vi "Initialize Attributes Core.vi"(8 "error in (no error)":errorcluster, 10 "Attribute Data":variant, 11 "BNT_DSCXYGraph in":refnum<class "BNT_DSCXYGraph.lvclass">) -> (0 "error out":errorcluster, 2 "MandatoryParameters":cluster{"Parameter":string, "found?":bool}[](array[cluster]), 3 "BNT_DSCXYGraph out":refnum<class "BNT_DSCXYGraph.lvclass">)   [LabVIEW 2018, in "BNT_DSCXYGraph.lvlib" / "BNT_DSCXYGraph.lvclass"]
doc: "Initialize object attribute.\n\nUnique resources should be allocated elsewhere!"
uses:
  BNT_DSCXYGraph.lvclass
  BNT_DSCXYGraph.lvclass/BNT_DSCXYGraph.ctl
  CSPP_Core/Actors/CSPP_GUIActor/CSPP_GUIActor.lvclass
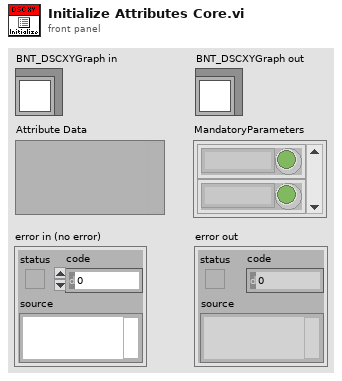
[diagram p1: front panel]
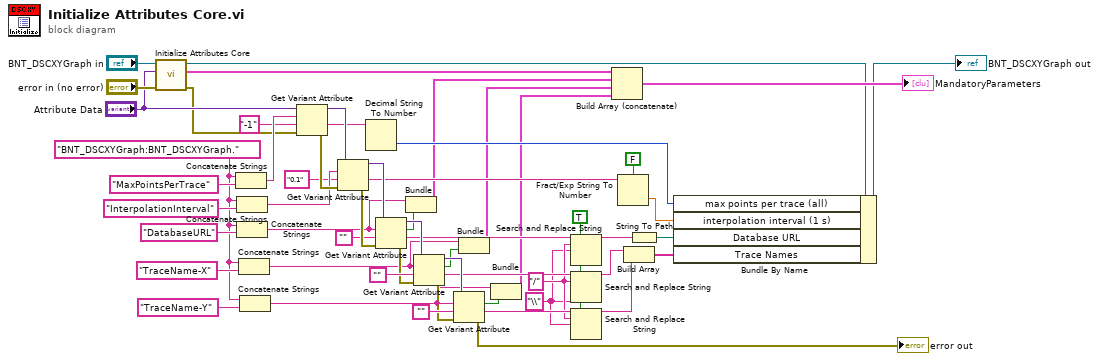
[diagram p0: block diagram]
diagram:
  w12 = TRUE ("replace all? (F)")
  w10 = "\\" ("replace string (\"\")")
  w11 = "/" ("search string")
  w41 = "BNT_DSCXYGraph:BNT_DSCXYGraph."
  n1 = call-parent "Initialize Attributes Core.vi"("error in (no error)"="error in (no error)", "Attribute Data"="Attribute Data", "CSPP_GUIActor in"="BNT_DSCXYGraph in") -> ("error out"=w47:errorcluster, "MandatoryParameters"=w48:cluster{"Parameter":string, "found?":bool}[], "CSPP_GUIActor out"=w20:refnum<class "BNT_DSCXYGraph.lvclass">)  [unwired: 6 in]
  n2 = Concatenate Strings(w41, "MaxPointsPerTrace" ("string")) -> (w53:string)
  n3 = Concatenate Strings(w41, "InterpolationInterval" ("string")) -> (w50:string)
  n4 = Concatenate Strings(w41, "DatabaseURL" ("string")) -> (w8:string)
  n5 = Concatenate Strings(w41, "TraceName-X" ("string")) -> (w6:string)
  n6 = Concatenate Strings(w41, "TraceName-Y" ("string")) -> (w2:string)
  n7 = Get Variant Attribute(Variant="Attribute Data", name=w53, default value (empty Variant)="-1" ("string"), error in=w47) -> (duplicate Variant=w52:variant, value=w25:string, error out=w51:errorcluster)  [unwired: 1 out]
  n8 = Get Variant Attribute(Variant=w52, name=w50, default value (empty Variant)="0.1" ("string"), error in=w51) -> (duplicate Variant=w38:variant, value=w23:string, error out=w37:errorcluster)  [unwired: 1 out]
  n9 = Decimal String To Number(string=w25) -> (number=w24:i32)  [unwired: 2 in, 1 out]
  n10 = Get Variant Attribute(Variant=w38, name=w8, default value (empty Variant)="", error in=w37) -> (duplicate Variant=w34:variant, found=w7:bool, value=w13:string, error out=w33:errorcluster)
  n11 = Bundle(w8, w7) -> (w9:cluster{string, bool})  [unwired: 1 in]
  n12 = Get Variant Attribute(Variant=w34, name=w6, default value (empty Variant)="", error in=w33) -> (duplicate Variant=w30:variant, found=w5:bool, value=w18:string, error out=w31:errorcluster)
  n13 = Get Variant Attribute(Variant=w30, name=w2, default value (empty Variant)="", error in=w31) -> (found=w1:bool, value=w16:string, error out=→"error out":errorcluster)  [unwired: 1 out]
  n14 = Bundle(w6, w5) -> (w4:cluster{string, bool})  [unwired: 1 in]
  n15 = Bundle(w2, w1) -> (w3:cluster{string, bool})  [unwired: 1 in]
  n16 = Search and Replace String(replace all?=w12, input string=w13, search string=w11, replace string=w10) -> (result string=w14:string)  [unwired: 4 in, 3 out]
  n17 = Search and Replace String(replace all?=w12, input string=w18, search string=w11, replace string=w10) -> (result string=w17:string)  [unwired: 4 in, 3 out]
  n18 = Search and Replace String(replace all?=w12, input string=w16, search string=w11, replace string=w10) -> (result string=w15:string)  [unwired: 4 in, 3 out]
  n19 = Build Array (concatenate)(w48, w9, w4, w3) -> (→"MandatoryParameters":cluster{"Parameter":string, "found?":bool}[])
  n20 = Fract/Exp String To Number(use system decimal point (T)=FALSE, string=w23) -> (number=w22:dbl)  [unwired: 2 in, 1 out]
  n21 = Build Array(w17, w15) -> (w26:string[])
  n22 = String To Path(string=w14) -> (path=w27:path)
  n23 = Bundle By Name(cluster=w20, "max points per trace (all)"=w24, "interpolation interval (1 s)"=w22, "Database URL"=w27, "Trace Names"=w26) -> (→"BNT_DSCXYGraph out":refnum<class "BNT_DSCXYGraph.lvclass">)
